vi "Read Attributes.vi"(11 "New UI Reference Msg":refnum<class "New UI Reference Msg.lvclass">) -> (2 "Payload":cluster{"VI Refnum":refnum<vi>, "Name":string})   [LabVIEW 2020, in "Chat Window Model.lvlib" / "New UI Reference Msg.lvclass"]
uses:
  New UI Reference Msg.lvclass
  New UI Reference Msg.lvclass/New UI Reference Msg.ctl
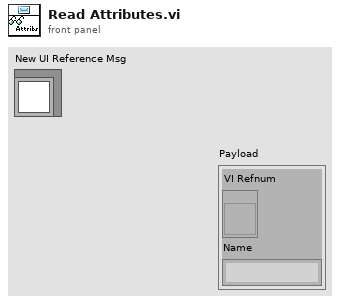
[diagram p1: front panel]
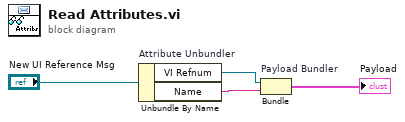
[diagram p0: block diagram]
diagram:
  n1 = Unbundle By Name "Attribute Unbundler"("New UI Reference Msg") -> ("VI Refnum"=w2:refnum<vi>, "Name"=w1:string)
  n2 = Bundle "Payload Bundler"("VI Refnum"=w2, "Name"=w1) -> (→"Payload":cluster{"VI Refnum":refnum<vi>, "Name":string})  [unwired: 1 in]
